vi "UnitTest-DeleteData.vi"(8 "error in":errorcluster) -> (0 "error out":errorcluster)   [LabVIEW 2014, in "TableLogger_CSV_Actor.lvlib" / "TableLogger_CSV_Actor.lvclass"]
uses:
  TableLogger_CSV_Actor.lvclass
  TableLogger_Actor/TableLoggerConfig.ctl
  TableLogger_Actor/TableLoggerTypes.ctl
  TableLogger_Actor/TableLoggerBackupConfig.ctl
  <vilib>/addons/_JKI Toolkits/Caraya/classes/Test/Test.lvclass
  <vilib>/addons/_JKI Toolkits/Caraya/classes/Assert/Assert.lvclass
  TableLogger_Actor/TableLogger_Actor.lvlib
panel:
  # "This example to check CSV Delete on Tablelogger"
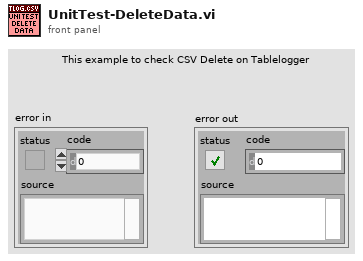
[diagram p1: front panel]
types:
  T1 = typedef "TableLogger_Actor.lvlib/TableLoggerConfig.ctl" = cluster{"TableLogger":T2, "DB File Path":path, "DB Backup Config":T3}
  T2 = typedef "TableLogger_Actor.lvlib/TableLoggerTypes.ctl" = enum16{"CSV Logger", "SQLite Logger"}
  T3 = typedef "TableLogger_Actor.lvlib/TableLoggerBackupConfig.ctl" = cluster{"Directory":path, "UTC Time Format":bool, "On Launch":bool, "Interval (Hours)":dbl, "Size Multiples (Bytes)":i32}
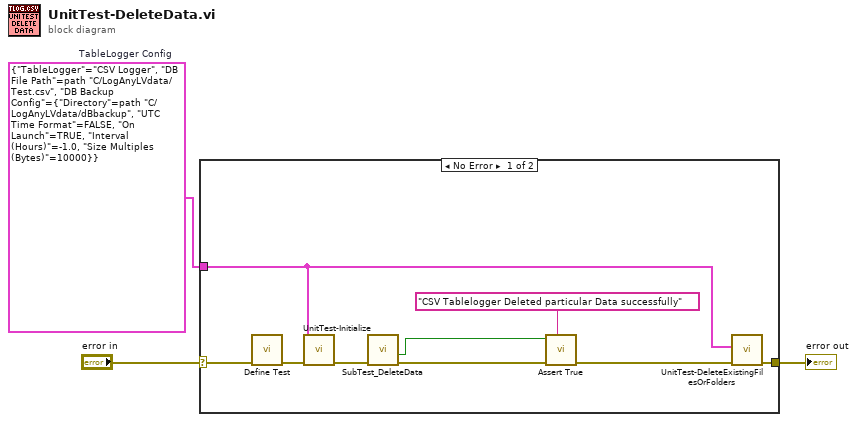
[diagram p0: block diagram]
diagram:
  w3 = T1 {"TableLogger"=enum."CSV Logger", "DB File Path"=path "C:/LogAnyLVdata/Test.csv", "DB Backup Config"={"Directory"=path "C:/LogAnyLVdata/dBbackup", "UTC Time Format"=FALSE, "On Launch"=TRUE, "Interval (Hours)"=-1.0, "Size Multiples (Bytes)"=10000}}  # TableLogger Config
  n1 = case shown="No Error" "error in" {
    selector: "error in" -> [w12 w13]
    tunnel: w3 -> [w9 _]
    tunnel: [w11 w13] -> w2
    frame No Error {
      n2 = call <vilib>:"Define Test.vi"("error in (no error)"=w12) -> ("error out"=w10:errorcluster)  [unwired: 10 in]
      n3 = call "UnitTest-Initialize.vi"("error in"=w10, "Config IN"=w9) -> ("error out"=w6:errorcluster)  [unwired: 7 in, 2 out]
      n4 = call "SubTest_DeleteData.vi"("error in (no error)"=w6) -> ("error out"=w5:errorcluster, "Deleted?T"=w4:bool)  [unwired: 9 in]
      n5 = call <vilib>:"Assert True.vi"("Label"="CSV Tablelogger Deleted particular Data successfully", "error in (no error)"=w5, "True?"=w4) -> ("error out"=w7:errorcluster)  [unwired: 8 in]
      n6 = call "UnitTest-DeleteExistingFilesOrFolders.vi"("error in (no error)"=w7, "Config IN"=w9) -> ("error out"=w11:errorcluster)  [unwired: 9 in]
    }
    frame Error {
    }
  }
  "error out" <- w2
